vi "Global Status bar event.vi"() -> ()   [LabVIEW 2013]
doc: "This is status bar global variable, that can be changed from anywhere to set message to status bar"
panel:
  in  "Global Status Bar event":refnum<user-event>
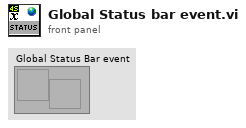
[diagram p1: front panel]
diagram:
